vi "Gray if True.vi"(1 "Checkbox":bool) -> (0 "Enabled":T1(ring))   [LabVIEW 2014, in "Endigit.lvlib"]
uses:
  Endigit.lvlib
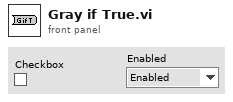
[diagram p1: front panel]
types:
  T1 = enum8{"Enabled", "Disabled", "Disabled and Grayed Out"}
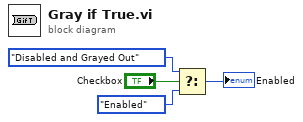
[diagram p0: block diagram]
diagram:
  n1 = Select(t=T1."Disabled and Grayed Out" ("Disabled"), s="Checkbox", f=T1."Enabled" ("Disabled")) -> (s? t:f=→"Enabled":T1)
